vi "Set Progress State.vi"(8 "error in (no error)":errorcluster, 10 "State (No Progress)":T1 items=["NoProgress"=0, "Indeterminate"=1, "Normal"=2, "Error"=4, "Paused"=8], 11 "Window Handle":refnum<k24>) -> (0 "error out":errorcluster, 3 "dup Window Handle":refnum<k24>)   [LabVIEW 2011, in "TaskbarProgressAPI.lvlib"]
doc: "Set the state of the Progress bar embedded in the Taskbar button of the Window referenced by the Window Handle.\n\nProgress bar States:\n- NoProgress = No progress is displayed.\n- Indeterminate = The progress is indeterminate (marquee).\n- Normal = Normal progress is displayed.\n- Error = An error occurred (red).\n- Paused = The operation is paused (yellow).\n\nPlease see the 'LabVIEW Taskbar Progress Bar API Example.vi' in the NI Example finder for details on how to use this VI."
uses:
  TaskbarProgressAPI.lvlib
  _TypeDefs/Progress State.ctl
  C:/Users/nlvanzwk/Dropbox/LabVIEW/LabVIEW Tools Network/LabVIEW Taskbar Progress Bar API/LabVIEW Taskbar Progress Bar API/Windows7Taskbar.dll
  Windows7Taskbar.dll
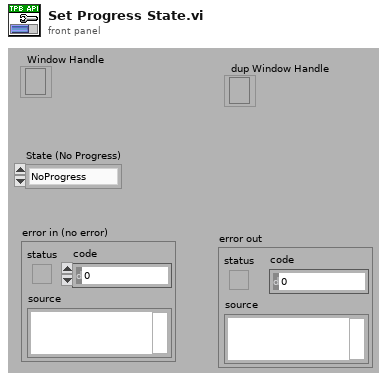
[diagram p1: front panel]
types:
  T1 = typedef "TaskbarProgressAPI.lvlib/Progress State.ctl" = i32
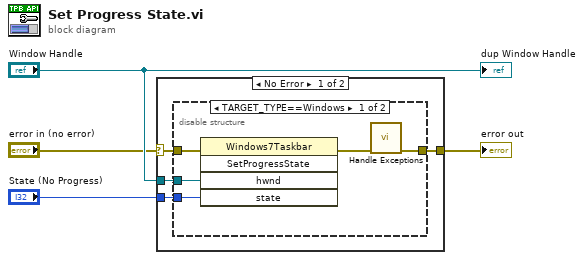
[diagram p0: block diagram]
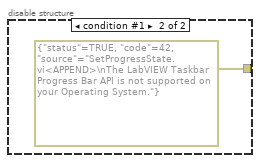
[diagram p2: hidden frame]
diagram:
  n1 = case shown="No Error" "error in (no error)" {
    selector: "error in (no error)" -> [w5 w15]
    tunnel: [w8 w15] -> w4
    tunnel: "Window Handle" -> [w7 _]
    tunnel: "State (No Progress)" -> [w6 _]
    frame No Error {
      n2 = disable-structure shown="TARGET_TYPE==Windows" {
        disable-tunnel: [w9 errorcluster {"status"=TRUE, "code"=42, "source"="SetProgressState.vi<APPEND>\nThe LabVIEW Taskbar Progress Bar API is not supported on your Operating System."} ("error out")] -> w8
        disable-tunnel: w7 -> [w13 _]
        disable-tunnel: w6 -> [w12 _]
        disable-tunnel: w5 -> [w11 _]
        frame condition #0 (active) {
          n3 = invoke class="Windows7Taskbar" method="SetProgressState"(error in=w11, "hwnd"=w13, "state"=w12) -> (error out=w10:errorcluster)  [unwired: 2 in, 4 out]
          n4 = call "Handle Exceptions.vi"("error in (no error)"=w10) -> ("error out"=w9:errorcluster)  [unwired: 10 in]
        }
        frame condition #1 {
        }
      }
    }
    frame Error {
    }
  }
  "error out" <- w4
  "dup Window Handle" <- "Window Handle"
